vi "Configure Trigger (NFC - Source).vi"(8 "error in (no error)":errorcluster, 9 "Enable Reverse Polarity (F: Disable)":bool, 10 "Trigger Source (0: Channel 1)":i32(ring) items=["Channel 1", "Channel 2", "Channel 3", "Channel 4"], 11 "VISA resource name":refnum<visa-resource-name>) -> (0 "error out":errorcluster, 3 "VISA resource name out":refnum<visa-resource-name>)   [LabVIEW 2015, in "Agilent 2000 3000 X-Series.lvlib"]
doc: "Configures the input waveform source for the NFC (Near Field Communication) trigger.\n\n<b>Note:</b>\nThis VI is only applicable for 3000T, 3000G, 4000 X-Series."
uses:
  Agilent 2000 3000 X-Series.lvlib
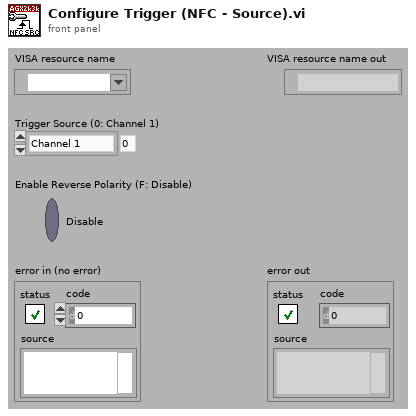
[diagram p1: front panel]
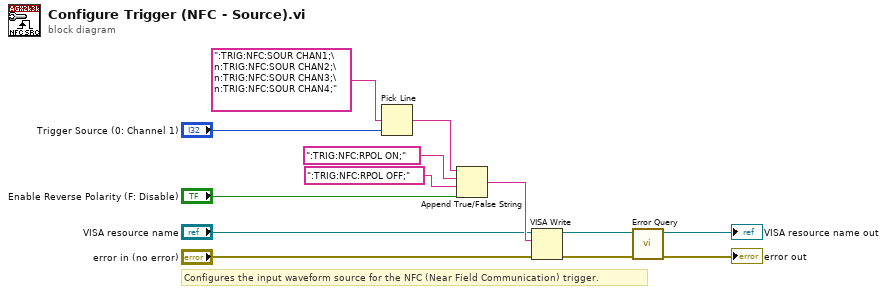
[diagram p0: block diagram]
diagram:
  # "Configures the input waveform source for the NFC (Near Field Communication) trigger."
  n1 = Pick Line(multi-line string=":TRIG:NFC:SOUR CHAN1;\n:TRIG:NFC:SOUR CHAN2;\n:TRIG:NFC:SOUR CHAN3;\n:TRIG:NFC:SOUR CHAN4;", line index="Trigger Source (0: Channel 1)") -> (output string=w11:string)  [unwired: 1 in]
  n2 = Append True/False String(1:"Enable Reverse Polarity (F: Disable)", 2:":TRIG:NFC:RPOL OFF;", 3:":TRIG:NFC:RPOL ON;", 4:w11) -> (0:w7:string)
  n3 = VISA Write(VISA resource name="VISA resource name", write buffer=w7, error in (no error)="error in (no error)") -> (VISA resource name out=w4:refnum<visa-resource-name>, error out=w3:errorcluster)  [unwired: 1 out]
  n4 = call "Error Query.vi"("error in (no error)"=w3, "VISA resource name"=w4) -> ("error out"=→"error out":errorcluster, "VISA resource name out"=→"VISA resource name out":refnum<visa-resource-name>)  [unwired: 6 in, 2 out]
